vi "Choreo_TrajectoryDifferential_Splits.vi"(11 "ChoreoTrajectoryDifferential":T1) -> (3 "splits":i32[](array[numeric]))   [LabVIEW 2019, in "ChoreoLib.lvlib"]
doc: "Returns the indices of the splits in the trajectory.\n\nInputs:\n -- ChoreoTrajectorySwerve - cluster - data cluster for this trajectory \n\nOutputs: \n -- Splits - integer array - the indices of the splits in the trajectory."
uses:
  ChoreoLib.lvlib
  TypeDef/ChoreoTrajectoryDifferential.ctl
  TypeDef/ChoreoDifferentialSample.ctl
  TypeDef/ChoreoEventMarker.ctl
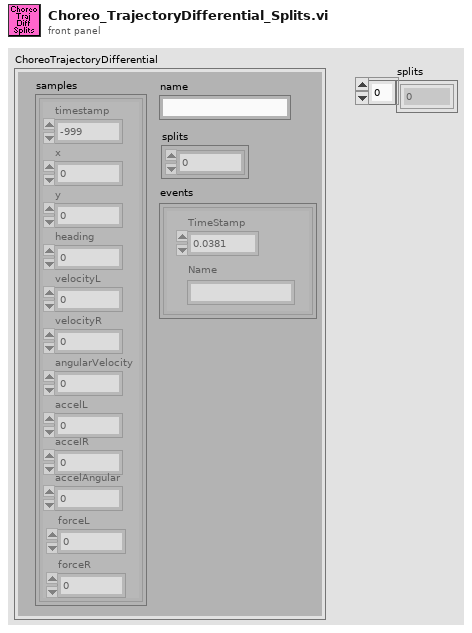
[diagram p1: front panel]
types:
  T1 = typedef "ChoreoLib.lvlib/ChoreoTrajectoryDifferential.ctl" = cluster{"name":string, "samples":T2[], "splits":i32[], "events":T3[]}
  T2 = typedef "ChoreoLib.lvlib/ChoreoDifferentialSample.ctl" = cluster{"timestamp":dbl, "x":dbl, "y":dbl, "heading":dbl, "velocityL":dbl, "velocityR":dbl, "angularVelocity":dbl, "accelL":dbl, "accelR":dbl, "accelAngular":dbl, "forceL":dbl, "forceR":dbl}
  T3 = typedef "ChoreoLib.lvlib/ChoreoEventMarker.ctl" = cluster{"TimeStamp":dbl, "Name":string}
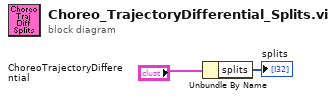
[diagram p0: block diagram]
diagram:
  n1 = Unbundle By Name("ChoreoTrajectoryDifferential") -> ("splits"=→"splits":i32[])
